vi "GetDataEventsForEquipment.vi"(8 "error in (no error)":errorcluster, 10 "equipment id":string, 11 "service":refnum<class "IcmMessageService.lvclass">) -> (0 "error out":errorcluster, 3 "DataEvents":T1[](array[typedef]))   [LabVIEW 2016]
doc: "Queries for data events containing data sets for an equipment node."
uses:
  <vilib>/addons/InsightCM/MessageBus/MessageService/IcmMessageService.lvclass
  <vilib>/addons/InsightCM/MessageBus/Base/controls/DataEventQueryParams.ctl
  <vilib>/addons/InsightCM/MessageBus/MessageLibrary/DataManagement/controls/DataManagementQueryEventsRequestBody.ctl
  <vilib>/addons/InsightCM/MessageBus/Base/controls/KeyValuePair.ctl
  <vilib>/addons/InsightCM/MessageBus/Base/controls/DataEvent.ctl
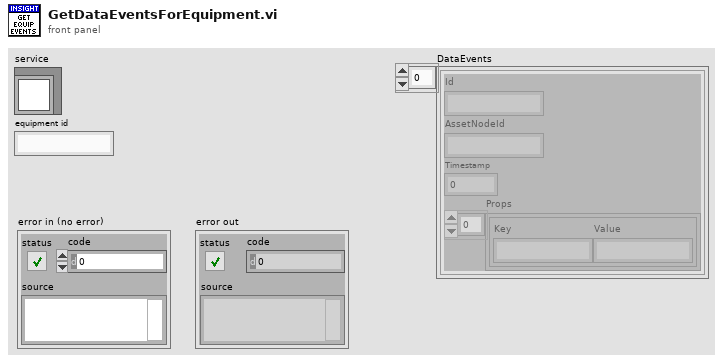
[diagram p1: front panel]
types:
  T1 = typedef "DataEvent.ctl" = cluster{"Id":string, "AssetNodeId":string, "Timestamp":i64, "Props":T2[]}
  T2 = typedef "KeyValuePair.ctl" = cluster{"Key":string, "Value":string}
  T3 = typedef "DataManagementQueryEventsRequestBody.ctl" = cluster{"AssetNodeId":string, "QueryParams":T4}
  T4 = typedef "DataEventQueryParams.ctl" = cluster{"StartTs":i64, "EndTs":i64, "OpState":string, "StreamsOnly":bool, "CommentsOnly":bool, "CommentSearch":string, "RetainOnly":bool, "Reason":string, "OrderBy":string, "OrderByDescending":string, "Skip":i32, "Take":i32, "HasDataSetsOnly":bool}
  T5 = typedef "Message.ctl" = cluster{"Header":T6, "Body":u8[]}
  T6 = typedef "MessageHeader.ctl" = cluster{"MessageName":string, "Timestamp":i64, "CorrelationId":string, "ContentType":string, "RoutingKey":string, "Properties":T2[]}
  T7 = typedef "DataManagementQueryEventsResponseBody.ctl" = cluster{"DataEvents":T1[], "TotalCount":i32}
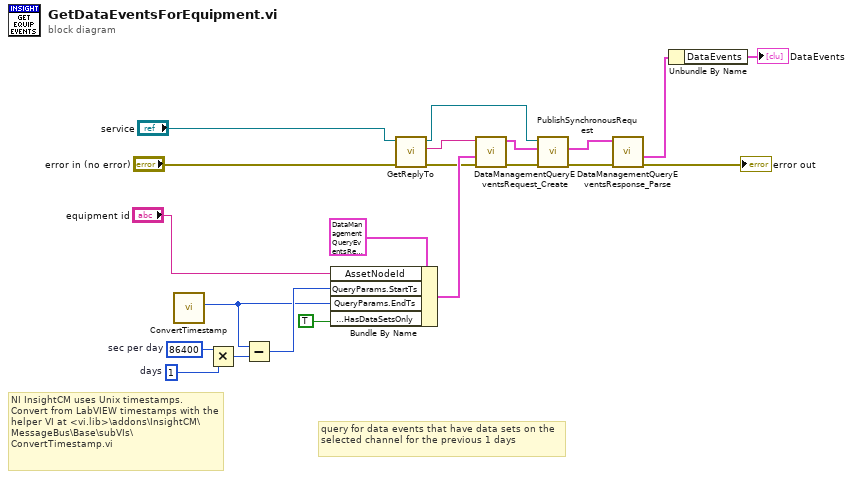
[diagram p0: block diagram]
diagram:
  w17 = 1  # days
  w18 = 86400  # sec per day
  # "NI InsightCM uses Unix timestamps. Convert from LabVIEW timestamps with the helper VI at <vi.lib>\\addons\\InsightCM\\MessageBus\\Base\\subVIs\\ConvertTimestamp.vi"
  # "query for data events that have data sets on the selected channel for the previous 1 days"
  n1 = call <vilib>:"ConvertTimestamp.vi"() -> ("Timestamp out"=w14:i64)  [unwired: 11 in]
  n2 = Multiply(x=w18, y=w17) -> (x*y=w16:i32)
  n3 = Subtract(x=w14, y=w16) -> (x-y=w15:i64)
  n4 = Bundle By Name(cluster=T3 {"AssetNodeId"="", "QueryParams"={"StartTs"=0, "EndTs"=0, "OpState"="", "StreamsOnly"=FALSE, "CommentsOnly"=FALSE, "CommentSearch"="", "RetainOnly"=FALSE, "Reason"="", "OrderBy"="", "OrderByDescending"="", "Skip"=0, "Take"=0, "HasDataSetsOnly"=FALSE}} ("Body"), "AssetNodeId"="equipment id", "QueryParams.StartTs"=w15, "QueryParams.EndTs"=w14, "QueryParams.HasDataSetsOnly"=TRUE) -> (w11:T3)
  n5 = call <vilib>:"GetReplyTo.vi"("error in (no error)"="error in (no error)", "service in"="service") -> ("error out"=w10:errorcluster, "reply to"=w7:string, "service out"=w21:refnum<class "IcmMessageService.lvclass">)  [unwired: 7 in]
  n6 = call <vilib>:"DataManagementQueryEventsRequest_Create.vi"("error in (no error)"=w10, "DataManagementQueryEventsRequest"=w11, "ReplyTo"=w7) -> ("error out"=w9:errorcluster, "Message"=w8:T5)  [unwired: 7 in]
  n7 = call <vilib>:"PublishSynchronousRequest.vi"("error in (no error)"=w9, "request"=w8, "service in"=w21) -> ("error out"=w6:errorcluster, "response"=w4:T5)  [unwired: 6 in, 1 out]
  n8 = call <vilib>:"DataManagementQueryEventsResponse_Parse.vi"("error in (no error)"=w6, "Message"=w4) -> ("error out"=→"error out":errorcluster, "Body"=w3:T7)  [unwired: 6 in, 2 out]
  n9 = Unbundle By Name(w3) -> ("DataEvents"=→"DataEvents":T1[])
